vi "2D Quadrature Formula Str Func.vi"(9 "data":variant, 10 "Y":dbl[](array[numeric]), 11 "X":dbl[](array[numeric])) -> (0 "error out":errorcluster, 3 "F(X,Y)":dbl[](array[numeric]))   [LabVIEW 2010, in "NI_AALPro.lvlib"]
uses:
  NI_AALPro.lvlib
  NI_Gmath.lvlib
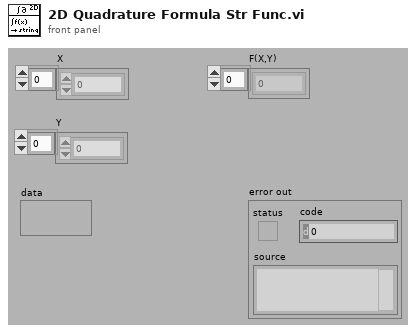
[diagram p1: front panel]
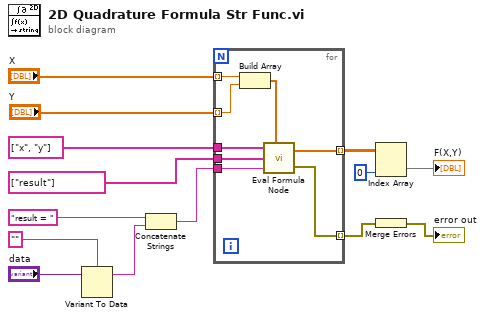
[diagram p0: block diagram]
diagram:
  n1 = Variant To Data(Variant="data", type="" ("string")) -> (data=w7:string)  [unwired: 1 in, 1 out]
  n2 = Concatenate Strings("result = " ("string"), w7) -> (w13:string)
  n3 = for {
    tunnel: w13 -> [w22]
    tunnel: string[] ["result"] ("Variables Output") -> [w21]
    tunnel: string[] ["x", "y"] ("Variables Output") -> [w20]
    tunnel: "X" -> [w19] mode=indexing
    tunnel: [w17] -> w4 mode=indexing
    tunnel: [w16] -> w5 mode=indexing
    tunnel: "Y" -> [w15] mode=indexing
    n4 = Build Array(w19, w15) -> (w18:dbl[])
    n5 = call "Eval Formula Node.vi"("Variables Input"=w20, "Input Values"=w18, "Variables Output"=w21, "formula"=w22) -> ("Output Values"=w17:dbl[], "error out"=w16:errorcluster)  [unwired: 1 in]
  }
  n6 = Index Array(array=w4, index (col)=0 ("disabled index (col)")) -> (element=→"F(X,Y)":dbl[])  [unwired: 1 in]
  n7 = Merge Errors(w5) -> (→"error out":errorcluster)
